vi "bcd-decade-counter.vi"() -> ()   [LabVIEW 2021]
panel:
  out "!Q":bool
  in  "CLK":bool
  in  "K 2":bool
  in  "J":bool
  out "Q":bool
  out "Clock Output":bool
  out "Elapsed mS":u32
  in  "Run Clock":bool
  in  "Step":bool
  in  "Clock Rate (Hz)":dbl
  in  "Stop Button":bool
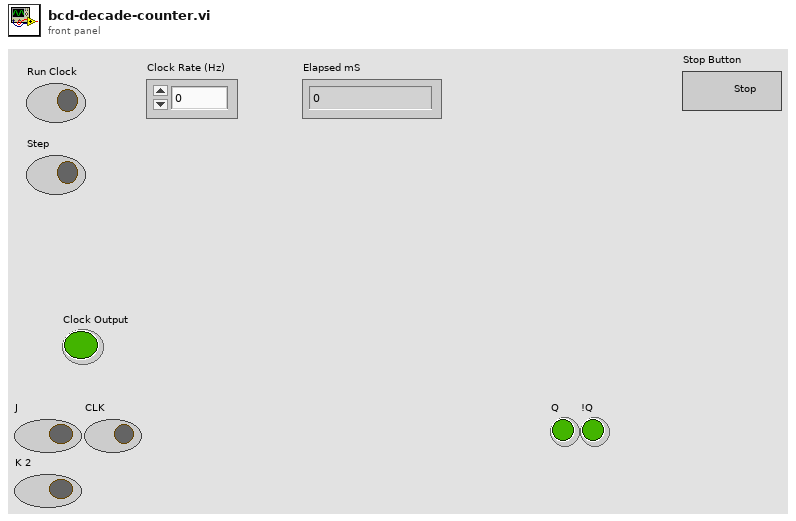
[diagram p1: front panel]
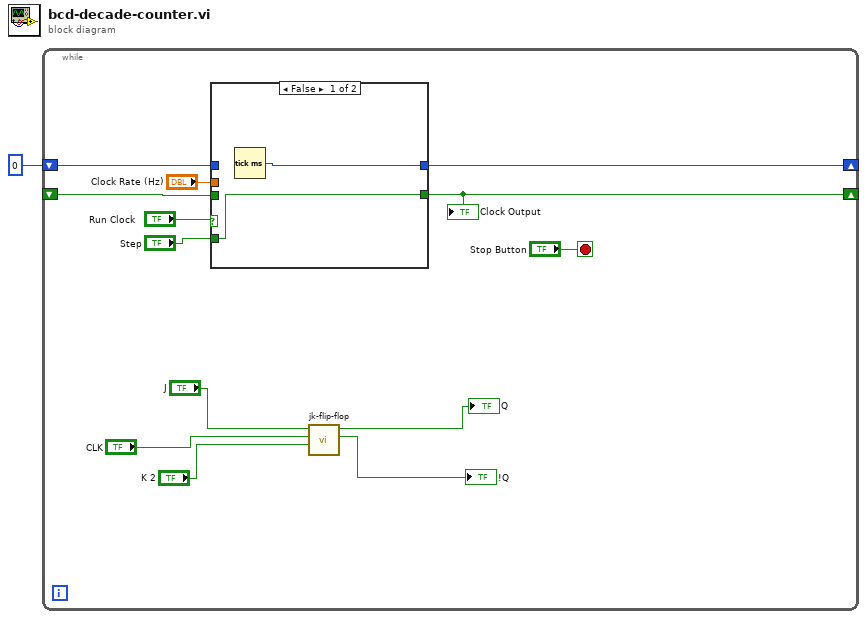
[diagram p0: block diagram]
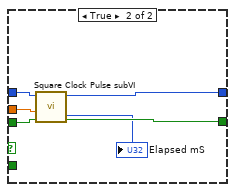
[diagram p2: hidden frame]
diagram:
  n1 = while {
    shift-right: [w10] -> _
    shift-left: u32 0 ("Last Event mS") -> [w9]
    shift-right: [w8] -> _
    shift-left: _ -> [w7]
    stop <- "Stop Button" stop-if-true
    n2 = case shown="False" "Run Clock" {
      tunnel: "Clock Rate (Hz)" -> [_ w22]
      tunnel: "Step" -> [w16 _]
      tunnel: [w15 w21] -> w10
      tunnel: w9 -> [_ w20]
      tunnel: [w16 w19] -> w8
      tunnel: w7 -> [_ w18]
      frame False {
        n3 = Tick Count (ms)() -> (millisecond timer value=w15:u32)
      }
      frame True {
        n4 = call "Square Clock Pulse subVI.vi"("Last Bool State"=w18, "Sample Rate (Hz)"=w22, "Last Event mS"=w20) -> ("Clock Output"=w19:bool, "Last Event mS"=w21:u32, "Elapsed mS"=→"Elapsed mS":u32)  [unwired: 5 in, 1 out]
      }
    }
    "Clock Output" <- w8
    n5 = call "jk-flip-flop.vi"("K in"="K 2", "CLK"="CLK", "J"="J") -> ("!Q"=→"!Q":bool, "Q"=→"Q":bool)  [unwired: 7 in]
  }
